vi "Handle.vi"(11 "Ex Queue Actor in":refnum<class "Ex Queue Actor.lvclass">) -> (2 "Destroy?":bool, 3 "Ex Queue Actor out":refnum<class "Ex Queue Actor.lvclass">)   [LabVIEW 2021, in "Ex Queue Actor.lvlib" / "Ex Queue Actor.lvclass"]
uses:
  Ex Queue Actor.lvclass
  Ex Queue Actor.lvclass/Ex Queue Actor.ctl
  Actor/Queue Actor/Queue Actor.lvclass
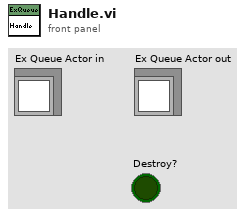
[diagram p1: front panel]
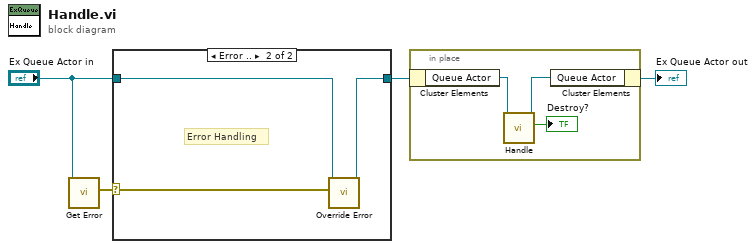
[diagram p0: block diagram]
diagram:
  n1 = call-dynamic "Get Error.vi"("Ex Queue Actor in"="Ex Queue Actor in") -> ("Error"=w1:errorcluster)  [unwired: 10 in]
  n2 = case shown="Error .." w1 {
    selector: w1 -> [_ w6]
    tunnel: "Ex Queue Actor in" -> [w5 w8]
    tunnel: [w5 w7] -> w3
    frame No Error {
    }
    frame Error {
      # "Error Handling"
      n3 = call-dynamic "Override Error.vi"("Error"=w6, "Ex Queue Actor in"=w8) -> ("Ex Queue Actor out"=w7:refnum<class "Ex Queue Actor.lvclass">)  [unwired: 9 in]
    }
  }
  n4 = in-place {
    n5 = in-place-cluster #1(w3) -> ("Queue Actor"=w11:refnum<class "Queue Actor.lvclass">)
    n6 = call-dynamic "Handle.vi"("Actor in"=w11) -> ("Destroy?"=→"Destroy?":bool, "Actor out"=w10:refnum<class "Queue Actor.lvclass">)  [unwired: 9 in]
    n7 = in-place-cluster #1("Queue Actor"=w10) -> (→"Ex Queue Actor out":refnum<class "Ex Queue Actor.lvclass">)
  }
